vi "Shutdown.vi"(8 "error in (no error)":errorcluster, 11 "Log_Engine in":refnum<class "Log_Engine.lvclass">) -> (0 "error out":errorcluster, 3 "Log_Engine out":refnum<class "Log_Engine.lvclass">)   [LabVIEW 2019, in "Log_Engine.lvclass"]
doc: "Developed by Kevin Thompson\nkevin@thompsonengineering.net\n\nCopyright 2018\nThompson Engineering, LLC"
uses:
  Log_Engine.lvclass
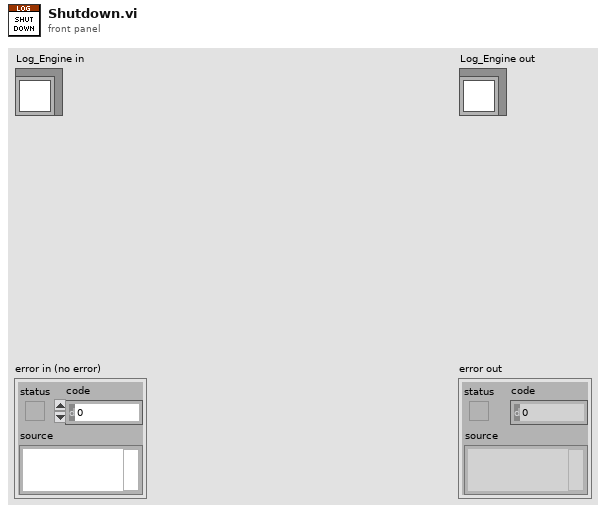
[diagram p1: front panel]
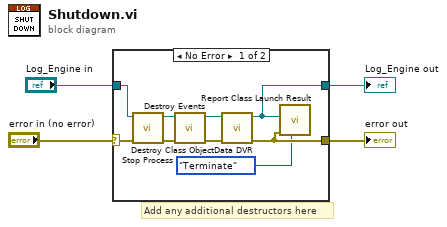
[diagram p0: block diagram]
diagram:
  # "Add any additional destructors here"
  n1 = case shown="No Error" "error in (no error)" {
    selector: "error in (no error)" -> [w5 w15]
    tunnel: [w8 w15] -> w3
    tunnel: [w9 w14] -> w1
    tunnel: "Log_Engine in" -> [w6 w14]
    frame No Error {
      n2 = call "Stop Process.vi"("error in (no error)"=w5, "Log_Engine in"=w6) -> ("error out"=w13:errorcluster, "Log_Engine out"=w12:refnum<class "Log_Engine.lvclass">)  [unwired: 8 in]
      n3 = call "Destroy Events.vi"("error in (no error)"=w13, "Log_Engine in"=w12) -> ("error out"=w11:errorcluster, "Log_Engine out"=w10:refnum<class "Log_Engine.lvclass">)  [unwired: 8 in]
      n4 = call "Destroy Class ObjectData DVR.vi"("error in (no error)"=w11, "Log_Engine in"=w10) -> ("error out"=w8:errorcluster, "Log_Engine out"=w9:refnum<class "Log_Engine.lvclass">)  [unwired: 8 in]
      n5 = call "Report Class Launch Result.vi"("Object"=w9, "error in (no error)"=w8, "Mode (Launch)"=enum16{"Launch", "Terminate"}."Terminate") -> ()  [unwired: 7 in, 1 out]
    }
    frame Error {
    }
  }
  "error out" <- w3
  "Log_Engine out" <- w1
